vi "Get Objects By ParentClass.vi"(8 "error in (no error)":errorcluster, 10 "parent class name":string="Constant", 11 "AllObjs[]":refnum<vi>[](array[refnum])) -> (3 "filtered objs":refnum<vi>[](array[refnum]))   [LabVIEW 2014]
doc: "Filter array of objects and returns only objects which are children of specified class name."
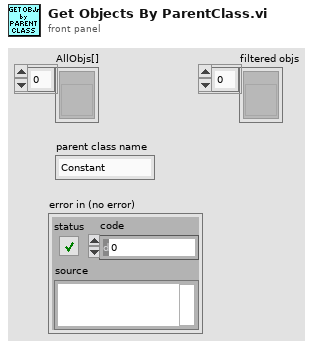
[diagram p1: front panel]
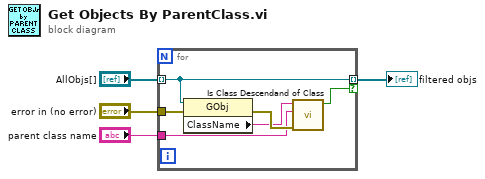
[diagram p0: block diagram]
diagram:
  n1 = for {
    tunnel: "AllObjs[]" -> [w9] mode=indexing
    tunnel: "error in (no error)" -> [w10]
    tunnel: [w9] -> w3 mode=indexing if=w5
    tunnel: "parent class name" -> [w6]
    n2 = property class="GObj"(reference=w9, error in=w10) -> (error out=w8:errorcluster, "ClassName"=w7:string)  [unwired: 1 out]
    n3 = call "Is Class Descendand of Class.vi"("Error In"=w8, "Parent ClassName"=w6, "ClassName"=w7) -> ("is Class descendant?"=w5:bool)  [unwired: 7 in, 1 out]
  }
  "filtered objs" <- w3
